vi "Introspection Core.vi"(8 "error in (no error)":errorcluster, 11 "BNT_ULx-MCSV-DOPWM in":refnum<class "BNT_ULx-MCSV-DOPWM.lvclass">) -> (0 "error out":errorcluster, 1 "CSPPMessages":refnum<class "Message.lvclass">[](array[class]), 2 "Class History":string[](array[string]), 3 "BNT_ULx-MCSV-DOPWM out":refnum<class "BNT_ULx-MCSV-DOPWM.lvclass">)   [LabVIEW 2020, in "BNT_ULx.lvlib" / "BNT_ULx-MCSV-DOPWM.lvclass"]
doc: "This vi delivers a list with all messages this actor reacts to. \n\nNote that all inherited classes have to overwrite it."
uses:
  BNT_ULx-MCSV-DOPWM.lvclass
  <vilib>/ActorFramework/Message/Message.lvclass
  BNT_ULx-MCSV-DOPWM Messages/Set Ratio Msg/Set Ratio Msg.lvclass
  C:/Program Files (x86)/National Instruments/LabVIEW 2020/vi.lib/ActorFramework/Message/Message.lvclass
  BNT_ULx-MCSV-DOPWM Messages/Set Ratios Msg/Set Ratios Msg.lvclass
  BNT_ULx-MCSV-DOPWM Messages/Set Delay Msg/Set Delay Msg.lvclass
  BNT_ULx-MCSV-DOPWM Messages/Set Delays Msg/Set Delays Msg.lvclass
  BNT_ULx-MCSV-DOPWM Messages/Set Length Msg/Set Length Msg.lvclass
  BNT_ULx-MCSV-DOPWM Messages/Set Lengths Msg/Set Lengths Msg.lvclass
  BNT_ULx-MCSV/BNT_ULx-MCSV.lvclass
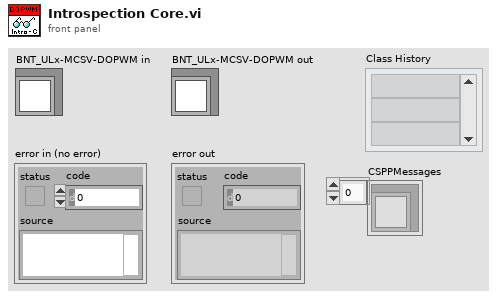
[diagram p1: front panel]
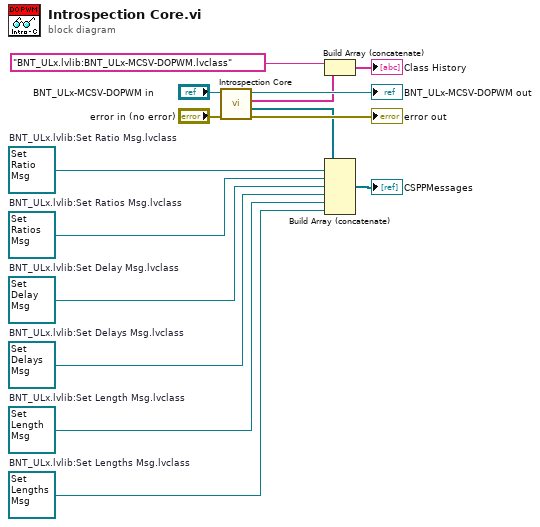
[diagram p0: block diagram]
diagram:
  w1 = refnum<class "Set Lengths Msg.lvclass"> refnum  # BNT_ULx.lvlib:Set Lengths Msg.lvclass
  w2 = refnum<class "Set Length Msg.lvclass"> refnum  # BNT_ULx.lvlib:Set Length Msg.lvclass
  w3 = refnum<class "Set Delays Msg.lvclass"> refnum  # BNT_ULx.lvlib:Set Delays Msg.lvclass
  w4 = refnum<class "Set Delay Msg.lvclass"> refnum  # BNT_ULx.lvlib:Set Delay Msg.lvclass
  w5 = refnum<class "Set Ratios Msg.lvclass"> refnum  # BNT_ULx.lvlib:Set Ratios Msg.lvclass
  w6 = refnum<class "Set Ratio Msg.lvclass"> refnum  # BNT_ULx.lvlib:Set Ratio Msg.lvclass
  n1 = call-parent "Introspection Core.vi"("error in (no error)"="error in (no error)", "BNT_ULx-MCSV in"="BNT_ULx-MCSV-DOPWM in") -> ("error out"=→"error out":errorcluster, "CSPPMessages"=w10:refnum<class "Message.lvclass">[], "Class History"=w9:string[], "BNT_ULx-MCSV out"=→"BNT_ULx-MCSV-DOPWM out":refnum<class "BNT_ULx-MCSV-DOPWM.lvclass">)  [unwired: 6 in]
  n2 = Build Array (concatenate)("BNT_ULx.lvlib:BNT_ULx-MCSV-DOPWM.lvclass", w9) -> (→"Class History":string[])
  n3 = Build Array (concatenate)(w10, w6, w5, w4, w3, w2, w1) -> (→"CSPPMessages":refnum<class "Message.lvclass">[])
